vi "Graph_Arrow.vi"(1 "magnitude":dbl=1.0, 2 "Heading":dbl step=15.0, 3 "plot data":T1) -> (0 "XY Graph":T2(graph))   [LabVIEW 2009]
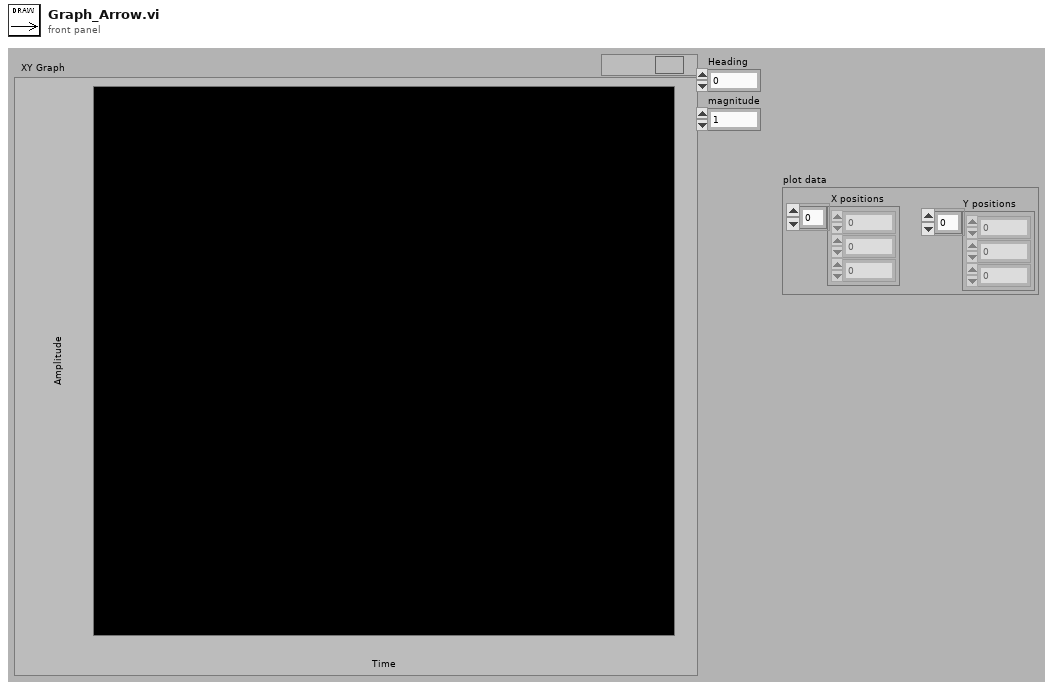
[diagram p1: front panel]
types:
  T1 = cluster{"X positions":dbl[], "Y positions":dbl[]}
  T2 = cluster{"initialized array":dbl[], "initialized array":dbl[]}[]
  T3 = cluster{"X positions":dbl[], "Y positions":dbl[]}[]
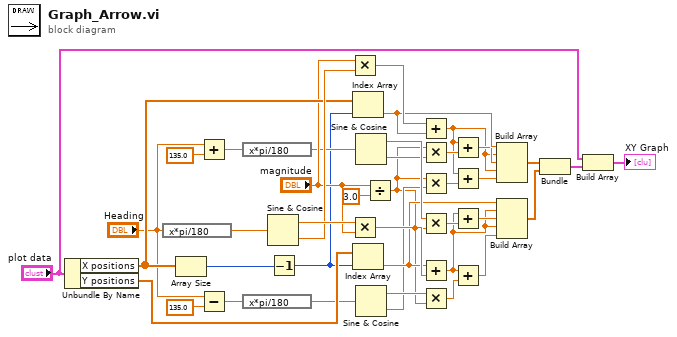
[diagram p0: block diagram]
diagram:
  n1 = Unbundle By Name("plot data") -> ("X positions"=w29:dbl[], "Y positions"=w30:dbl[])
  n2 = expression code="x*pi/180"("Heading") -> (w39:dbl)
  n3 = Array Size(array=w29) -> (size(s)=w17:i32)
  n4 = Add(x="Heading", y=135.0) -> (x+y=w25:dbl)
  n5 = Subtract(x="Heading", y=135.0) -> (x-y=w12:dbl)
  n6 = expression code="x*pi/180"(w25) -> (w24:dbl)
  n7 = expression code="x*pi/180"(w12) -> (w13:dbl)
  n8 = Sine & Cosine(0:w39) -> (1:w38:dbl, 2:w37:dbl)
  n9 = Decrement(x=w17) -> (x-1=w16:i32)
  n10 = Multiply(x="magnitude", y=w37) -> (x*y=w33:dbl)
  n11 = Multiply(x=w38, y="magnitude") -> (x*y=w32:dbl)
  n12 = Index Array(array=w29, index=w16) -> (element=w19:dbl)
  n13 = Index Array(array=w30, index=w16) -> (element=w18:dbl)
  n14 = Sine & Cosine(0:w24) -> (1:w23:dbl, 2:w22:dbl)
  n15 = Sine & Cosine(0:w13) -> (1:w10:dbl, 2:w9:dbl)
  n16 = Divide(x="magnitude", y=3.0) -> (x/y=w8:dbl)
  n17 = Add(x=w33, y=w19) -> (x+y=w6:dbl)
  n18 = Multiply(x=w8, y=w22) -> (x*y=w20:dbl)
  n19 = Multiply(x=w8, y=w9) -> (x*y=w5:dbl)
  n20 = Multiply(x=w23, y=w8) -> (x*y=w21:dbl)
  n21 = Add(x=w18, y=w32) -> (x+y=w3:dbl)
  n22 = Multiply(x=w10, y=w8) -> (x*y=w4:dbl)
  n23 = Add(x=w6, y=w20) -> (x+y=w14:dbl)
  n24 = Add(x=w6, y=w5) -> (x+y=w2:dbl)
  n25 = Add(x=w3, y=w21) -> (x+y=w15:dbl)
  n26 = Add(x=w3, y=w4) -> (x+y=w1:dbl)
  n27 = Build Array(w19, w6, w14, w6, w2) -> (w36:dbl[])
  n28 = Build Array(w18, w3, w15, w3, w1) -> (w35:dbl[])
  n29 = Bundle(w36, w35) -> (w34:cluster{dbl[], dbl[]})  [unwired: 1 in]
  n30 = Build Array("plot data", w34) -> (→"XY Graph":T3)
